vi "PMT_plus_Kinesis_plus_Keithley.vi"() -> ()   [LabVIEW 2022 SP3]
uses:
  <vilib>/Utility/file.llb/Write Delimited Spreadsheet (string).vi
  <vilib>/Analysis/1siggen.llb/Ramp Pattern by Delta.vi
  <vilib>/Utility/file.llb/Write Delimited Spreadsheet (DBL).vi
  C:/Users/Public/OneDrive/Desktop/PMT program/SampleCodeLabView/Kinesis_with_LabVIEW_Examples_LV12 - v3/ThorLabs.MotionControl.KCube.DCServoCLI.dll
  Kinesis_with_LabVIEW_Examples_LV12 - v3/ThorLabs.MotionControl.KCube.DCServoCLI.dll
  <vilib>/Analysis/NI_AALBase.lvlib
  C:/Users/Public/OneDrive/Desktop/PMT program/SampleCodeLabView/Kinesis_with_LabVIEW_Examples_LV12 - v3/Thorlabs.MotionControl.Controls.dll
  Kinesis_with_LabVIEW_Examples_LV12 - v3/Thorlabs.MotionControl.Controls.dll
  test_save_lv22/Close.vi/Close Folder/Users/Public/OneDrive/Desktop/Keithley_2450_2470_1_4_0_LV2015_NewReadme2_2450-LV2015-1.4.0/Keithley 2450/Keithley 2450.lvlib
  D:/Download/Keithley 24XX/Keithley 24XX Folder/D/Download/Keithley 24XX/Keithley 24XX.lvlib
panel:
  out "current 2410":dbl format="%e"
  in  "top: 2450\nbottom: 2410":bool
  in  "VISA resource name 2410":refnum<visa-resource-name>="GPIB1::16::INSTR"
  in  "wait for cur meas":u32=100
  out "XY Graph":cluster{dbl[], dbl[]}(graph)
  out "mean":dbl=49.0
  out "standard deviation":dbl
  out "OLD":bool
  out "data":u32[](array[numeric])=[49, 49]
  out "Actual Voltage":dbl
  out "current":dbl=2.5622937e-12 format="%e"
  out "error out":errorcluster
  out "Set Voltage":dbl
  in  "VISA resource name 2450":refnum<visa-resource-name>="GPIB0::1::INSTR"
  in  "error in (no error)":errorcluster
  out "Serial Configuration":T1={"Baud Rate"=9600, "Parity"=0, "Data Bits"=8, "Stop Bits"=10, "Flow Control"=0} {"Flow Control" items=["None", "XON/XOFF", "RTS/CTS", "XON/XOFF & RTS/CTS", "DTR/DSR", "XON/XOFF & DTR/DSR"]; "Stop Bits" items=["1.0"=10, "1.5"=15, "2.0"=20]; "Data Bits" items=["7"=7, "8"=8]; "Parity" items=["None", "Odd", "Even", "Mark", "Space"]; "Baud Rate" items=["300"=300, "600"=600, "1200"=1200, "2400"=2400, "4800"=4800, "9600"=9600, "19200"=19200]}
  in  "Num Current Meas":i32=20
  in  "Source Limit Level (0.1)":dbl=1e-08
  in  "wait for move (ms)":u32=14000
  out "Handle Number":i32=173123648
  in  "Start V":dbl format="%#_13g"
  in  "End V":dbl=0.2 format="%#_13g"
  in  "Step Size (V)":dbl=0.1 format="%#_13g"
  in  "Path":path=path "C:/Users/Public/OneDrive/Desktop/test.txt"
  in  "Use PMT?":bool=TRUE
  in  "Loop?":bool
  in  "KCubeDCServoControl":refnum<k24>(container)
  in  "Motor Controller SerialNumber":string="27268499"
  in  "quarter waveplate p1":dbl=142.0 format="%#_13g"
  in  "quarter waveplate p2":dbl=232.0 format="%#_13g"
  out "PC":dbl caption="Current Rotation Position"
  out "DB":u32[](array[numeric])=[49, 0, 0, 0, 0, 0, 0, 0, 0, 0, 0, 0, 0, 0, 0, 0]
  out "Overload":i32
  out "Gate Number":i32=1
  out "Num Gates Read":i32=2
  out "Gate Time Read":i32=100 caption="Gate time Read"
  out "Num Gates Set":i32=20
  out "Gate Time Set":i32=300
  out "PowerD":i32 caption="Power\nRead Data"
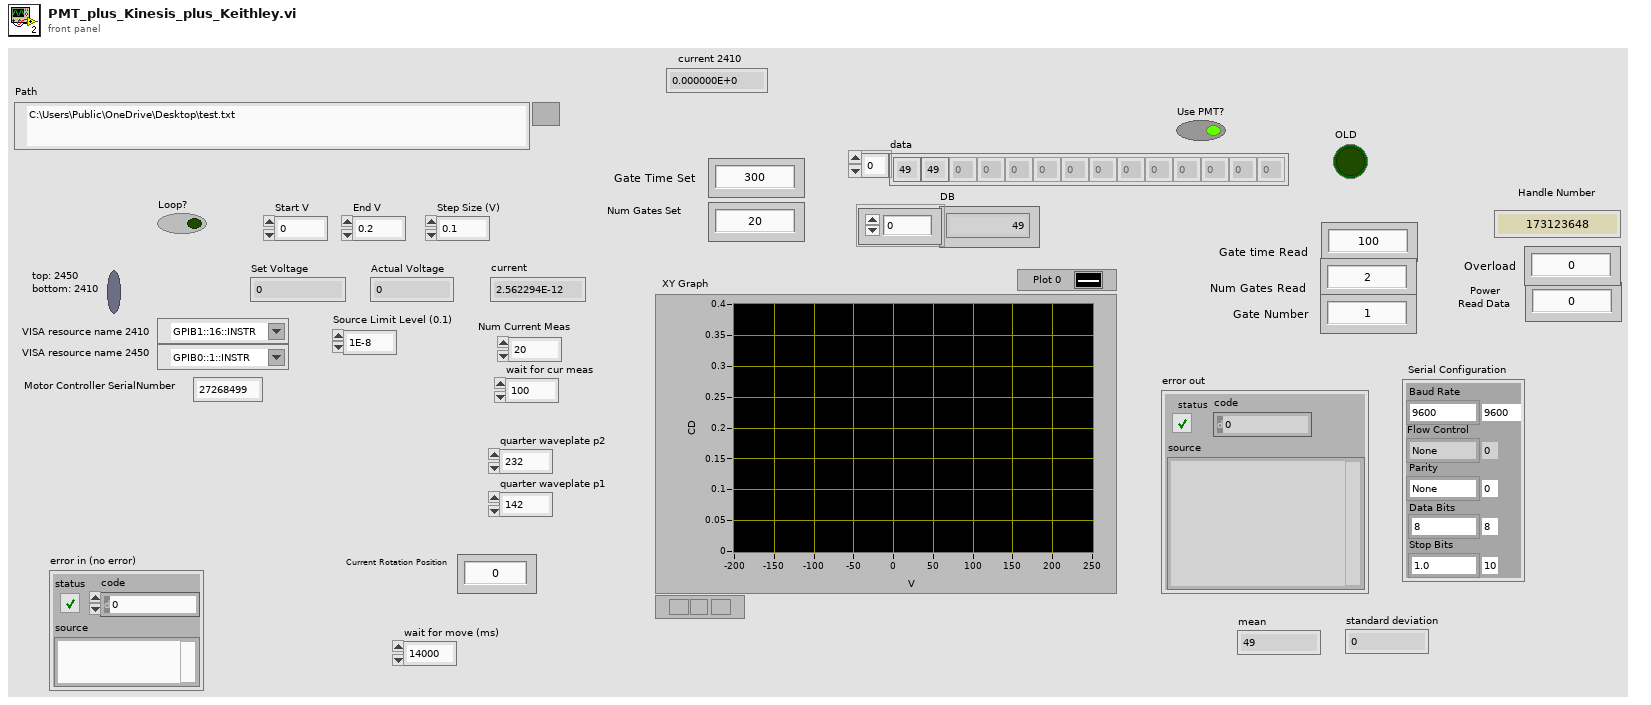
[diagram p1: front panel]
types:
  T1 = cluster{"Baud Rate":u32, "Parity":u16, "Data Bits":u16, "Stop Bits":u16, "Flow Control":u16}
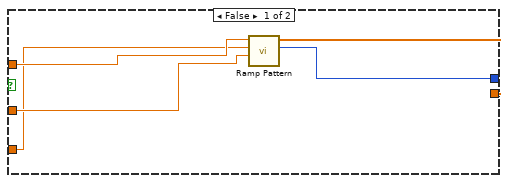
[diagram p2: hidden frame]
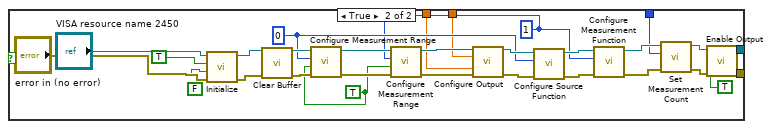
[diagram p3: hidden frame]
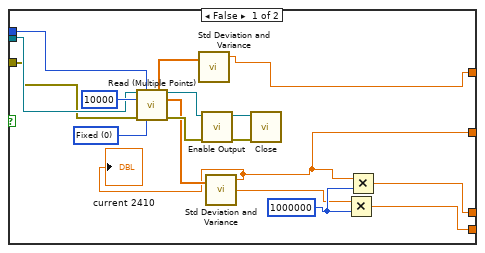
[diagram p4: hidden frame]
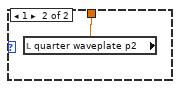
[diagram p5: hidden frame]
diagram:
  n1 = flat-sequence {
    tunnel: [w47] -> w22
    tunnel: [w38] -> w21
    tunnel: ["Path"] -> w20
    tunnel: [w37] -> w19
    tunnel: [w26] -> w18
    tunnel: [w23] -> w17
    tunnel: w22 -> [w83]
    tunnel: [w83] -> w16
    tunnel: w21 -> [w82]
    tunnel: [w82] -> w15
    tunnel: w20 -> [w81]
    tunnel: [w81] -> w14
    tunnel: w19 -> [w80]
    tunnel: [w80] -> w13
    tunnel: [w79] -> w12
    tunnel: w18 -> [w79]
    tunnel: ["wait for move (ms)"] -> w11
    tunnel: [w77] -> w10
    tunnel: w17 -> [w77]
    tunnel: w16 -> [w94]
    tunnel: [w94] -> w9
    tunnel: w15 -> [w93]
    tunnel: [w93] -> w8
    tunnel: w14 -> [w92]
    tunnel: [w92] -> w7
    tunnel: w13 -> [w91]
    tunnel: [w91] -> w6
    tunnel: w12 -> [w90]
    tunnel: [w89] -> w5
    tunnel: [w85] -> w4
    tunnel: w11 -> [w85]
    tunnel: [w84] -> w3
    tunnel: w10 -> [w84]
    tunnel: w9 -> [w106]
    tunnel: w8 -> [w105]
    tunnel: [w104] -> w2
    tunnel: w7 -> [w103]
    tunnel: w6 -> [w98]
    tunnel: w5 -> [w95]
    tunnel: w4 -> [w97]
    tunnel: w3 -> [w96]
    tunnel: [w95] -> w1
    tunnel: w2 -> [w644]
    tunnel: w1 -> [w637]
    frame #0 {
      # "open PMT and turn on power"
      n2 = local write "quarter waveplate p2"("quarter waveplate p2") -> ()
      n3 = local write "quarter waveplate p1"("quarter waveplate p1") -> ()
      n4 = call "Open.vi"("Serial Number"="30430219") -> ("Handle Number"=w51:i32)  [unwired: 9 in, 1 out]
      "Handle Number" <- w51
      n5 = case shown="True" "Loop?" {
        tunnel: "Start V" -> [w58 w69]
        tunnel: "End V" -> [w57 w67]
        tunnel: [w60 w66] -> w37
        tunnel: [w61 w65] -> w38
        tunnel: "Step Size (V)" -> [w59 w63]
        frame False {
          n6 = call-poly <vilib>:"Ramp Pattern.vi"("start"=w58, "end"=w57, "delta"=w59) -> ("samples"=w61:i32, "Ramp Pattern"=w60:dbl[])  [unwired: 6 in, 1 out]
        }
        frame True {
          w64 = -1.0
          n7 = Multiply(x=w63, y=w64) -> (x*y=w62:dbl)
          n8 = Multiply(x=w67, y=w64) -> (x*y=w68:dbl)
          n9 = call-poly <vilib>:"Ramp Pattern.vi"("start"=w69, "end"=w67, "delta"=w63) -> ("samples"=w73:i32, "Ramp Pattern"=w70:dbl[])  [unwired: 6 in, 1 out]
          n10 = call-poly <vilib>:"Ramp Pattern.vi"("start"=w68, "end"=w69, "delta"=w63) -> ("samples"=w76:i32, "Ramp Pattern"=w72:dbl[])  [unwired: 6 in, 1 out]
          n11 = call-poly <vilib>:"Ramp Pattern.vi"("start"=w67, "end"=w68, "delta"=w62) -> ("samples"=w74:i32, "Ramp Pattern"=w71:dbl[])  [unwired: 6 in, 1 out]
          n12 = Add(x=w73, y=w74) -> (x+y=w75:i32)
          n13 = Build Array (concatenate)(w70, w71, w72) -> (w66:dbl[])
          n14 = Add(x=w75, y=w76) -> (x+y=w65:i32)
        }
      }
      n15 = call "Read HV.vi"("handle"=w51) -> ("HV out"=w50:i32, "handle out"=w54:i32)  [unwired: 8 in, 1 out]
      n16 = Boolean To (0,1)(Boolean="Use PMT?") -> (0, 1=w52:i16)
      n17 = local write "PowerD"(w50) -> ()
      n18 = To Long Integer(number=w52) -> (32bit integer=w53:i32)
      n19 = call "Set HV.vi"("HV"=w53, "handle"=w54) -> ("handle out"=w56:i32)  [unwired: 8 in, 1 out]
      n20 = property class="KCubeDCServoControl"(reference="KCubeDCServoControl", "SerialNumber"="Motor Controller SerialNumber") -> (reference out=w36:refnum<k24>)  [unwired: 1 in, 1 out]
      n21 = invoke class="KCubeDCServoControl" method="CreateDevice"(reference=w36) -> (reference out=w33:refnum<k24>)  [unwired: 2 in, 2 out]
      n22 = property class="KCubeDCServoControl"(reference=w33) -> ("Device"=w23:refnum<k24>)  [unwired: 1 in, 2 out]
      n23 = call "Read HV.vi"("handle"=w56) -> ("HV out"=w55:i32, "handle out"=w47:i32)  [unwired: 8 in, 1 out]
      n24 = local write "PowerD"(w55) -> ()
      n25 = invoke class="KCubeDCServo" method="GetPositionCounter"(reference=w23) -> (reference out=w29:refnum<k24>, "GetPositionCounter"=w32:i32)  [unwired: 2 in, 1 out]
      n26 = Divide(x=w32, y=1919.6418578623338) -> (x/y=w30:dbl)
      n27 = local write "PC"(w30) -> ()
      n28 = invoke class="KCubeDCServo" method="SetMoveAbsolutePosition"(reference=w29, "position"="quarter waveplate p1") -> (reference out=w28:refnum<k24>)  [unwired: 2 in, 3 out]
      n29 = invoke class="KCubeDCServo" method="MoveAbsolute"(reference=w28, "waitTimeout"=0) -> (reference out=w26:refnum<k24>)  [unwired: 2 in, 3 out]
      n30 = Build Array("# SetVoltage(V) ActualVoltage(V) CountsMeancirc1 Countsmeancirc2 CountsStdcirc1 CountsStdcirc2 Current(uA) CurrentStd(uA) CircularDichroism") -> (w42:string[])
      n31 = call-poly <vilib>:"Write Delimited Spreadsheet.vi"("file path (dialog if empty)"="Path", "1D data"=w42, "append to file? (new file:F)"=TRUE) -> ()  [unwired: 11 in, 2 out]
    }
    frame #1 {
      n32 = Wait (ms)(milliseconds to wait="wait for move (ms)") -> ()  [unwired: 1 out]
    }
    frame #2 {
      n33 = invoke class="KCubeDCServo" method="GetPositionCounter"(reference=w90) -> (reference out=w89:refnum<k24>, "GetPositionCounter"=w87:i32)  [unwired: 2 in, 1 out]
      n34 = Divide(x=w87, y=1919.6418578623338) -> (x/y=w86:dbl)
      n35 = local write "PC"(w86) -> ()
    }
    frame #3 {
      w101 = 0
      w102 = 0
      n36 = Initialize Array(w102, w102) -> (w99:i32[])
      n37 = Initialize Array(w101, w101) -> (w100:i32[])
      n38 = for {
        N: w105 -> [_]
        tunnel: w98 -> [w162] mode=indexing
        tunnel: w106 -> [w138]
        tunnel: [w161] -> w104
        tunnel: w103 -> [w134]
        shift-right: [w152] -> _
        shift-left: w99 -> [w157]
        shift-right: [w153] -> _
        shift-left: w100 -> [w156]
        tunnel: w95 -> [w130]
        tunnel: w97 -> [w126]
        tunnel: w96 -> [w112]
        n39 = flat-sequence {
          tunnel: w156 -> [w169]
          tunnel: w157 -> [w174]
          tunnel: w162 -> [w168]
          tunnel: [w168] -> w151
          tunnel: [w174] -> w149
          tunnel: [w169] -> w147
          tunnel: [w167] -> w145
          tunnel: [w166] -> w143
          tunnel: ["Num Current Meas"] -> w139
          tunnel: w138 -> [w173]
          tunnel: [w173] -> w135
          tunnel: w134 -> [w172]
          tunnel: [w172] -> w131
          tunnel: w130 -> [w171]
          tunnel: [w171] -> w127
          tunnel: w112 -> [w170]
          tunnel: [w170] -> w110
          tunnel: ["top: 2450\nbottom: 2410"] -> w107
          tunnel: w151 -> [w233]
          tunnel: [w233] -> w150
          tunnel: w149 -> [w232]
          tunnel: [w232] -> w148
          tunnel: w147 -> [w231]
          tunnel: [w231] -> w146
          tunnel: w145 -> [w230]
          tunnel: [w230] -> w144
          tunnel: w143 -> [w229]
          tunnel: [w229] -> w142
          tunnel: [w228] -> w140
          tunnel: w139 -> [w228]
          tunnel: [w226] -> w136
          tunnel: w135 -> [w226]
          tunnel: [w225] -> w132
          tunnel: w131 -> [w225]
          tunnel: [w224] -> w128
          tunnel: w127 -> [w224]
          tunnel: [w223] -> w111
          tunnel: w110 -> [w223]
          tunnel: [w222] -> w108
          tunnel: w107 -> [w222]
          tunnel: [w248] -> w160
          tunnel: [w235] -> w159
          tunnel: [w241] -> w158
          tunnel: [w247] -> w155
          tunnel: [w246] -> w154
          tunnel: w150 -> [w248]
          tunnel: w148 -> [w247]
          tunnel: w146 -> [w246]
          tunnel: w144 -> [w244]
          tunnel: w142 -> [w245]
          tunnel: [w242] -> w141
          tunnel: w140 -> [w243]
          tunnel: [w239] -> w137
          tunnel: w136 -> [w239]
          tunnel: [w238] -> w133
          tunnel: w132 -> [w238]
          tunnel: [w237] -> w129
          tunnel: w128 -> [w237]
          tunnel: w111 -> [w236]
          tunnel: [w236] -> w109
          tunnel: w108 -> [w234]
          tunnel: w160 -> [w314]
          tunnel: w159 -> [w313]
          tunnel: w158 -> [w312]
          tunnel: w155 -> [w311]
          tunnel: w154 -> [w310]
          tunnel: [w315] -> w125
          tunnel: [w309] -> w122
          tunnel: w141 -> [w308]
          tunnel: w137 -> [w307]
          tunnel: w133 -> [w303]
          tunnel: w129 -> [w305]
          tunnel: w126 -> [w304]
          tunnel: [w303] -> w120
          tunnel: [w302] -> w119
          tunnel: [w297] -> w118
          tunnel: [w296] -> w117
          tunnel: [w295] -> w116
          tunnel: [w294] -> w115
          tunnel: [w293] -> w114
          tunnel: [w292] -> w113
          tunnel: w109 -> [w291]
          tunnel: w125 -> [w631]
          tunnel: [w631] -> w124
          tunnel: [w622] -> w123
          tunnel: w122 -> [w613]
          tunnel: [w612] -> w121
          tunnel: w120 -> [w629]
          tunnel: w119 -> [w627]
          tunnel: w118 -> [w610]
          tunnel: w117 -> [w620]
          tunnel: w116 -> [w626]
          tunnel: w115 -> [w625]
          tunnel: w114 -> [w623]
          tunnel: w113 -> [w621]
          tunnel: [w633] -> w152
          tunnel: [w634] -> w153
          tunnel: [w635] -> w161
          tunnel: w124 -> [w635]
          tunnel: w123 -> [w634]
          tunnel: w121 -> [w633]
          frame #0 {
            n40 = case shown="False" "top: 2450\nbottom: 2410" {
              tunnel: w168 -> [w175 w198]
              tunnel: [w177 w196] -> w167
              tunnel: [w178 w195] -> w166
              tunnel: "Num Current Meas" -> [_ w194]
              tunnel: "Source Limit Level (0.1)" -> [w176 w193]
              frame False {
                w180 = TRUE
                w181 = u16 0 items=["Voltage", "Current"] ("Source Mode  (0: Voltage)")
                w182 = u16 1 items=["Volts", "Current", "Resistance"] ("Function (0: Volts)")
                w183 = u16 0 items=["Volts", "Current", "Resistance"] ("Function (0: Volts)")
                n41 = call "Initialize.vi"("Reset (True)"=FALSE, "VISA resource name"="VISA resource name 2410") -> ("error out"=w190:errorcluster, "VISA resource name out"=w191:refnum<visa-resource-name>)  [unwired: 8 in]
                n42 = call "Configure Measurement.vi"("error in (no error)"=w190, "Enable Auto Range (T:Enable)"=w180, "Function (0: Volts)"=w183, "VISA resource name"=w191) -> ("error out"=w189:errorcluster, "VISA resource name out"=w188:refnum<visa-resource-name>)  [unwired: 6 in]
                n43 = call "Configure Measurement.vi"("error in (no error)"=w189, "Enable Auto Range (T:Enable)"=w180, "Function (0: Volts)"=w182, "VISA resource name"=w188) -> ("error out"=w186:errorcluster, "VISA resource name out"=w187:refnum<visa-resource-name>)  [unwired: 6 in]
                n44 = call "Configure Output.vi"("Source Mode  (0: Voltage)"=w181, "error in (no error)"=w186, "Compliance  Level (0.1)"=w176, "Output Level (0)"=w175, "VISA resource name"=w187) -> ("error out"=w184:errorcluster, "VISA resource name out"=w185:refnum<visa-resource-name>)  [unwired: 5 in]
                n45 = call "Enable Output.vi"("error in (no error)"=w184, "VISA resource name"=w185) -> ("error out"=w177:errorcluster, "VISA resource name out"=w178:refnum<visa-resource-name>)  [unwired: 8 in]
              }
              frame True {
                w197 = 1
                w200 = 0
                w201 = TRUE
                n46 = call "Initialize.vi"("error in (no error)"="error in (no error)", "Reset (True)"=FALSE, "ID Query (True)"=TRUE, "VISA resource name"="VISA resource name 2450") -> ("error out"=w221:errorcluster, "VISA resource name out"=w218:refnum<visa-resource-name>)  [unwired: 6 in]
                n47 = call "Clear Buffer.vi"("VISA resource name"=w218, "error in (no error)"=w221) -> ("VISA resource name out"=w213:refnum<visa-resource-name>, "error out"=w212:errorcluster)  [unwired: 12 in]
                n48 = call "Configure Measurement Range.vi"("error in (no error)"=w212, "Enable Auto Range (T:Enable)"=w201, "Function (0: Volts)"=w200, "VISA resource name"=w213) -> ("error out"=w204:errorcluster, "VISA resource name out"=w205:refnum<visa-resource-name>)  [unwired: 6 in]
                n49 = call "Configure Measurement Range.vi"("error in (no error)"=w204, "Enable Auto Range (T:Enable)"=w201, "Function (0: Volts)"=w197, "VISA resource name"=w205) -> ("error out"=w208:errorcluster, "VISA resource name out"=w211:refnum<visa-resource-name>)  [unwired: 6 in]
                n50 = call "Configure Output.vi"("VISA resource name"=w211, "Source Level (0)"=w198, "Source Limit Level (0.1)"=w193, "error in (no error)"=w208) -> ("VISA resource name out"=w210:refnum<visa-resource-name>, "error out"=w207:errorcluster)  [unwired: 10 in]
                n51 = call "Configure Source Function.vi"("error in (no error)"=w207, "Function (0: Volts)"=w200, "VISA resource name"=w210) -> ("error out"=w206:errorcluster, "VISA resource name out"=w209:refnum<visa-resource-name>)  [unwired: 7 in]
                n52 = call "Configure Measurement Function.vi"("error in (no error)"=w206, "Function (0: Volts)"=w197, "VISA resource name"=w209) -> ("error out"=w217:errorcluster, "VISA resource name out"=w214:refnum<visa-resource-name>)  [unwired: 7 in]
                n53 = call "Set Measurement Count.vi"("error in (no error)"=w217, "Measurement Count (1)"=w194, "VISA resource name"=w214) -> ("error out"=w216:errorcluster, "VISA resource name out"=w215:refnum<visa-resource-name>)  [unwired: 7 in]
                n54 = call "Enable Output.vi"("error in (no error)"=w216, "Enable Output (T: Enable)"=TRUE, "VISA resource name"=w215) -> ("error out"=w196:errorcluster, "VISA resource name out"=w195:refnum<visa-resource-name>)  [unwired: 7 in]
              }
            }
            "Set Voltage" <- w168
          }
          frame #1 {
            n55 = Wait (ms)(milliseconds to wait="wait for cur meas") -> ()  [unwired: 1 out]
          }
          frame #2 {
            n56 = case shown="True" w234 {
              tunnel: w245 -> [w251 w290]
              tunnel: w244 -> [w249 w289]
              tunnel: w243 -> [w250 w288]
              tunnel: [w252 w287] -> w242
              tunnel: [w253 w286] -> w241
              tunnel: [w254 w271] -> w240
              tunnel: [w257 w266] -> w235
              frame False {
                w256 = 1000000
                w265 = u16 0 items=["Fixed", "Sweep", "List"] ("Output Mode (0: Fixed)")
                n57 = call "Read (Multiple Points).vi"("VISA resource name"=w251, "Sample Count (1)"=w250, "Timeout (10000 ms)"=10000, "error in (no error)"=w249, "Output Mode (0: Fixed)"=w265) -> ("Voltage"=w258:sgl[], "VISA resource name out"=w263:refnum<visa-resource-name>, "Current"=w259:sgl[], "error out"=w260:errorcluster)  [unwired: 4 in, 3 out]
                n58 = call <vilib>:"Std Deviation and Variance.vi"("X"=w258) -> ("mean"=w257:dbl)  [unwired: 1 in, 2 out]
                n59 = call "Enable Output.vi"("error in (no error)"=w260, "VISA resource name"=w263) -> ("error out"=w261:errorcluster, "VISA resource name out"=w262:refnum<visa-resource-name>)  [unwired: 8 in]
                n60 = call <vilib>:"Std Deviation and Variance.vi"("X"=w259) -> ("mean"=w254:dbl, "standard deviation"=w255:dbl)  [unwired: 1 in, 1 out]
                "current 2410" <- w254
                n61 = call "Close.vi"("error in (no error)"=w261, "VISA resource name"=w262) -> ()  [unwired: 9 in, 1 out]
                n62 = Multiply(x=w255, y=w256) -> (x*y=w252:dbl)
                n63 = Multiply(x=w254, y=w256) -> (x*y=w253:dbl)
              }
              frame True {
                w270 = 1000000
                n64 = call "Make Reading and Store in Buffer.vi"("VISA resource name"=w290, "error in (no error)"=w289) -> ("VISA resource name out"=w282:refnum<visa-resource-name>, "error out"=w281:errorcluster)  [unwired: 12 in]
                n65 = call "Read (Multiple Points).vi"("VISA resource name"=w282, "Start Index (1)"=u32 1, "End Index (1)"=w288, "error in (no error)"=w281) -> ("VISA resource name out"=w274:refnum<visa-resource-name>, "Data out"=w279:string, "error out"=w273:errorcluster)  [unwired: 9 in]
                n66 = Spreadsheet String To Array(delimiter (Tab)=",", format string="%s", spreadsheet string=w279, array type (2D Dbl)=dbl[] []) -> (array=w275:dbl[])
                n67 = call "Get Source Level.vi"("error in (no error)"=w273, "VISA resource name"=w274) -> ("error out"=w284:errorcluster, "Voltage Level Out"=w266:dbl, "VISA resource name out"=w285:refnum<visa-resource-name>)  [unwired: 6 in, 1 out]
                n68 = call <vilib>:"Std Deviation and Variance.vi"("X"=w275) -> ("mean"=w271:dbl, "standard deviation"=w272:dbl)  [unwired: 1 in, 1 out]
                n69 = call "Enable Output.vi"("error in (no error)"=w284, "Enable Output (T: Enable)"=TRUE, "VISA resource name"=w285) -> ("error out"=w267:errorcluster, "VISA resource name out"=w268:refnum<visa-resource-name>)  [unwired: 7 in]
                n70 = Multiply(x=w272, y=w270) -> (x*y=w287:dbl)
                n71 = Multiply(x=w271, y=w270) -> (x*y=w286:dbl)
                n72 = call "Close.vi"("error in (no error)"=w267, "VISA resource name"=w268) -> ("error out"=→"error out":errorcluster)  [unwired: 9 in]
              }
            }
            "current" <- w240
            "Actual Voltage" <- w235
          }
          frame #3 {
            w299 = 0
            w301 = 0
            n73 = Initialize Array(w301, w301) -> (w300:i32[])
            n74 = Initialize Array(w299, w299) -> (w298:i32[])
            n75 = for {
              N: 2 -> [_]
              tunnel: w314 -> [w425]
              tunnel: w313 -> [w424]
              tunnel: w312 -> [w423]
              tunnel: w311 -> [w345]
              tunnel: w310 -> [w422]
              tunnel: [w421] -> w309
              tunnel: w308 -> [w420]
              shift-right: [w426] -> w315
              shift-left: w307 -> [w419]
              tunnel: w305 -> [w357]
              tunnel: w304 -> [w356]
              tunnel: [w346] -> w302
              shift-right: [w324] -> w297
              shift-left: w300 -> [w344]
              shift-right: [w323] -> w296
              shift-left: w298 -> [w334]
              tunnel: [w322] -> w295
              tunnel: [w321] -> w294
              tunnel: [w320] -> w293
              tunnel: [w319] -> w292
              tunnel: w291 -> [w318]
              i -> [w355]
              (unwired) "# SetVoltage2450(V) ActualVoltage2450(V) CountsMean CountsStd Current2450(uA) Current2450Std(uA)"
              # "- actual voltage array\n- actual voltage current\n- set voltage current\n-  current current\n- current std current"
              n76 = flat-sequence {
                tunnel: [w438] -> w371
                tunnel: [w436] -> w369
                tunnel: [w437] -> w367
                tunnel: w425 -> [w438]
                tunnel: w424 -> [w437]
                tunnel: w423 -> [w436]
                tunnel: w345 -> [w435]
                tunnel: [w435] -> w365
                tunnel: w422 -> [w434]
                tunnel: [w434] -> w363
                tunnel: w420 -> [w433]
                tunnel: [w433] -> w361
                tunnel: w419 -> [w432]
                tunnel: [w432] -> w359
                tunnel: w357 -> [_]
                tunnel: w355 -> [w430]
                tunnel: w344 -> [w429]
                tunnel: [w429] -> w340
                tunnel: w334 -> [w428]
                tunnel: [w428] -> w327
                tunnel: w318 -> [w427]
                tunnel: [w427] -> w317
                tunnel: w371 -> [w452]
                tunnel: [w452] -> w370
                tunnel: w369 -> [w451]
                tunnel: [w451] -> w368
                tunnel: w367 -> [w450]
                tunnel: [w450] -> w366
                tunnel: w365 -> [w449]
                tunnel: [w449] -> w364
                tunnel: w363 -> [w448]
                tunnel: [w448] -> w362
                tunnel: w361 -> [w447]
                tunnel: [w447] -> w360
                tunnel: w359 -> [w446]
                tunnel: [w446] -> w358
                tunnel: [w444] -> w341
                tunnel: w340 -> [w444]
                tunnel: [w443] -> w328
                tunnel: w327 -> [w443]
                tunnel: w317 -> [w442]
                tunnel: [w441] -> w316
                tunnel: [w460] -> w418
                tunnel: [w466] -> w417
                tunnel: w370 -> [w466]
                tunnel: [w465] -> w416
                tunnel: w368 -> [w465]
                tunnel: [w464] -> w415
                tunnel: w366 -> [w464]
                tunnel: [w463] -> w414
                tunnel: w364 -> [w463]
                tunnel: [w462] -> w413
                tunnel: w362 -> [w462]
                tunnel: [w461] -> w412
                tunnel: w360 -> [w461]
                tunnel: w358 -> [w460]
                tunnel: w356 -> [w459]
                tunnel: [w458] -> w342
                tunnel: w341 -> [w458]
                tunnel: [w457] -> w329
                tunnel: w328 -> [w457]
                tunnel: w316 -> [w453]
                tunnel: w418 -> [w481]
                tunnel: [w476] -> w411
                tunnel: [w474] -> w410
                tunnel: w417 -> [w474]
                tunnel: [w473] -> w409
                tunnel: w416 -> [w473]
                tunnel: [w472] -> w408
                tunnel: w415 -> [w472]
                tunnel: [w471] -> w407
                tunnel: w414 -> [w471]
                tunnel: [w470] -> w406
                tunnel: w413 -> [w470]
                tunnel: [w469] -> w405
                tunnel: w412 -> [w469]
                tunnel: [w468] -> w343
                tunnel: w342 -> [w468]
                tunnel: [w467] -> w330
                tunnel: w329 -> [w467]
                tunnel: [w492] -> w404
                tunnel: w411 -> [w494]
                tunnel: [w489] -> w403
                tunnel: w410 -> [w489]
                tunnel: w409 -> [w488]
                tunnel: [w488] -> w402
                tunnel: [w487] -> w401
                tunnel: w408 -> [w487]
                tunnel: [w486] -> w400
                tunnel: w407 -> [w486]
                tunnel: [w485] -> w399
                tunnel: w406 -> [w485]
                tunnel: [w484] -> w398
                tunnel: w405 -> [w484]
                tunnel: w343 -> [w483]
                tunnel: [w483] -> w337
                tunnel: [w482] -> w331
                tunnel: w330 -> [w482]
                tunnel: w404 -> [w509]
                tunnel: [w509] -> w397
                tunnel: [w505] -> w396
                tunnel: [w505] -> w395
                tunnel: [w504] -> w394
                tunnel: w403 -> [w504]
                tunnel: [w503] -> w393
                tunnel: w402 -> [w503]
                tunnel: w401 -> [w502]
                tunnel: [w502] -> w392
                tunnel: [w501] -> w391
                tunnel: w400 -> [w501]
                tunnel: [w500] -> w390
                tunnel: w399 -> [w500]
                tunnel: w398 -> [w499]
                tunnel: [w499] -> w389
                tunnel: [w498] -> w338
                tunnel: w337 -> [w498]
                tunnel: [w497] -> w332
                tunnel: w331 -> [w497]
                tunnel: w397 -> [w524]
                tunnel: [w520] -> w388
                tunnel: w396 -> [w519]
                tunnel: w395 -> [w518]
                tunnel: [w519] -> w387
                tunnel: [w518] -> w386
                tunnel: w394 -> [w517]
                tunnel: [w517] -> w385
                tunnel: [w516] -> w384
                tunnel: w393 -> [w516]
                tunnel: [w515] -> w383
                tunnel: w392 -> [w515]
                tunnel: [w514] -> w382
                tunnel: w391 -> [w514]
                tunnel: [w513] -> w381
                tunnel: w390 -> [w513]
                tunnel: [w512] -> w380
                tunnel: w389 -> [w512]
                tunnel: [w511] -> w339
                tunnel: w338 -> [w511]
                tunnel: [w510] -> w333
                tunnel: w332 -> [w510]
                tunnel: [w539] -> w379
                tunnel: w388 -> [w538]
                tunnel: w387 -> [w537]
                tunnel: w386 -> [w536]
                tunnel: [w535] -> w378
                tunnel: [w532] -> w377
                tunnel: w385 -> [w532]
                tunnel: [w531] -> w376
                tunnel: w384 -> [w531]
                tunnel: w383 -> [w530]
                tunnel: [w530] -> w375
                tunnel: [w529] -> w374
                tunnel: w382 -> [w529]
                tunnel: [w528] -> w373
                tunnel: w381 -> [w528]
                tunnel: [w527] -> w372
                tunnel: w380 -> [w527]
                tunnel: w339 -> [w526]
                tunnel: [w526] -> w336
                tunnel: w333 -> [w525]
                tunnel: [w525] -> w326
                tunnel: w379 -> [w595]
                tunnel: [w594] -> w353
                tunnel: [w593] -> w354
                tunnel: w378 -> [w593]
                tunnel: w377 -> [w592]
                tunnel: [w592] -> w352
                tunnel: [w591] -> w351
                tunnel: w376 -> [w591]
                tunnel: [w590] -> w350
                tunnel: w375 -> [w590]
                tunnel: [w589] -> w349
                tunnel: w374 -> [w589]
                tunnel: w373 -> [w588]
                tunnel: [w588] -> w348
                tunnel: [w587] -> w347
                tunnel: w372 -> [w587]
                tunnel: w336 -> [w586]
                tunnel: [w586] -> w335
                tunnel: w326 -> [w585]
                tunnel: [w585] -> w325
                tunnel: [w609] -> w426
                tunnel: w353 -> [w609]
                tunnel: w352 -> [w607]
                tunnel: w351 -> [w601]
                tunnel: w350 -> [w599]
                tunnel: w349 -> [w596]
                tunnel: w348 -> [w600]
                tunnel: [w596] -> w421
                tunnel: w347 -> [w598]
                tunnel: w354 -> [w608]
                tunnel: [w607] -> w346
                tunnel: w335 -> [w606]
                tunnel: w325 -> [w605]
                tunnel: [w603] -> w324
                tunnel: [w602] -> w323
                tunnel: [w601] -> w322
                tunnel: [w598] -> w321
                tunnel: [w600] -> w320
                tunnel: [w599] -> w319
                frame #0 {
                  n77 = case shown="0, Default" w430 {
                    tunnel: [w439 w440] -> w431
                    frame 0, Default {
                      n78 = local read "quarter waveplate p1"() -> (w439:dbl)
                    }
                    frame 1 {
                      n79 = local read "quarter waveplate p2"() -> (w440:dbl)
                    }
                  }
                  n80 = invoke class="KCubeDCServo" method="SetMoveAbsolutePosition"(reference=w427, "position"=w431) -> ()  [unwired: 2 in, 4 out]
                }
                frame #1 {
                  n81 = invoke class="KCubeDCServo" method="MoveAbsolute"(reference=w442, "waitTimeout"=0) -> (reference out=w441:refnum<k24>)  [unwired: 2 in, 3 out]
                }
                frame #2 {
                  n82 = Wait (ms)(milliseconds to wait=w459) -> ()  [unwired: 1 out]
                  n83 = invoke class="KCubeDCServo" method="GetPositionCounter"(reference=w453) -> ("GetPositionCounter"=w455:i32)  [unwired: 2 in, 2 out]
                  n84 = Divide(x=w455, y=1919.6418578623338) -> (x/y=w454:dbl)
                  n85 = local write "PC"(w454) -> ()
                }
                frame #3 {
                  # "set gate time"
                  n86 = local read "Gate Time Set"() -> (w478:i32)
                  n87 = Wait (ms)(milliseconds to wait=u32 200) -> ()  [unwired: 1 out]
                  n88 = To Long Integer(number=w478) -> (32bit integer=w479:i32)
                  n89 = call "Set IT.vi"("IT"=w479, "handle"=w481) -> ("handle out"=w480:i32)  [unwired: 8 in, 1 out]
                  n90 = call "Read IT.vi"("handle"=w480) -> ("IT out"=w477:i32, "handle out"=w476:i32)  [unwired: 8 in, 1 out]
                  n91 = local write "Gate Time Read"(w477) -> ()
                }
                frame #4 {
                  # "set number of gates"
                  n92 = local read "Num Gates Set"() -> (w496:i32)
                  n93 = Wait (ms)(milliseconds to wait=u32 200) -> ()  [unwired: 1 out]
                  n94 = To Long Integer(number=w496) -> (32bit integer=w495:i32)
                  n95 = call "Set RN.vi"("RN"=w495, "handle"=w494) -> ("handle out"=w493:i32)  [unwired: 8 in, 1 out]
                  n96 = call "Read RN.vi"("handle"=w493) -> ("RN out"=w491:i32, "handle out"=w492:i32)  [unwired: 8 in, 1 out]
                  n97 = local write "Num Gates Read"(w491) -> ()
                }
                frame #5 {
                  # "gate number data"
                  # "count data"
                  n98 = local write "Gate Number"(0) -> ()
                  n99 = Initialize Array(u32 0, 0 ("次元サイズ")) -> (w505:u32[])
                }
                frame #6 {
                  n100 = Boolean To (0,1)(Boolean=TRUE ("Correction")) -> (0, 1=w523:i16)
                  n101 = To Long Integer(number=w523) -> (32bit integer=w522:i32)
                  n102 = call "Count Start.vi"("Correction"=w522, "handle"=w524) -> ("handle out"=w520:i32)  [unwired: 8 in, 1 out]
                }
                frame #7 {
                  n103 = local read "Num Gates Read"() -> (w534:i32)
                  n104 = for {
                    N: w534 -> [_]
                    shift-right: [w540] -> w535
                    shift-left: w537 -> [w548]
                    shift-right: [w544] -> _
                    shift-left: w536 -> [w547]
                    tunnel: w538 -> [w549]
                    tunnel: [w550] -> w539
                    tunnel: [w540] -> w533
                    n105 = flat-sequence {
                      tunnel: [w560] -> w554
                      tunnel: [w559] -> w545
                      tunnel: [w558] -> w542
                      tunnel: w549 -> [w560]
                      tunnel: w548 -> [w559]
                      tunnel: w547 -> [w558]
                      tunnel: [w571] -> w553
                      tunnel: w554 -> [w570]
                      tunnel: [w565] -> w552
                      tunnel: [w564] -> w551
                      tunnel: [w563] -> w546
                      tunnel: w545 -> [w563]
                      tunnel: [w562] -> w543
                      tunnel: w542 -> [w562]
                      tunnel: [w561] -> w541
                      tunnel: w553 -> [w584]
                      tunnel: w552 -> [w579]
                      tunnel: w551 -> [w578]
                      tunnel: w546 -> [w576]
                      tunnel: w543 -> [w575]
                      tunnel: w541 -> [w574]
                      tunnel: [w584] -> w550
                      tunnel: [w577] -> w540
                      tunnel: [w572] -> w544
                      frame #0 {
                        n106 = Initialize Array(u32 0, 16 ("次元サイズ")) -> (w555:u32[])
                        n107 = local write "DB"(w555) -> ()
                      }
                      frame #1 {
                        # "read data"
                        n108 = local read "Gate Number"() -> (w569:i32)
                        n109 = local read "Overload"() -> (w568:i32)
                        n110 = local read "DB"() -> (w566:u32[])
                        n111 = call "Read Data.vi"("OLD"=w568, "DataBuf"=w566, "GateNum"=w569, "handle"=w570) -> ("OLD out"=w567:i32, "DataBuf out"=w564:u32[], "GateNum out"=w561:i32, "handle out"=w571:i32, "function return"=w565:u32)  [unwired: 3 in]
                        n112 = local write "Gate Number"(w561) -> ()
                        n113 = local write "DB"(w564) -> ()
                        n114 = local write "Overload"(w567) -> ()
                      }
                      frame #2 {
                        # "Pickup Tans Data!"
                        n115 = To Long Integer(number=w579) -> (32bit integer=w580:i32)
                        n116 = Build Array(w574) -> (w573:i32[])
                        n117 = local read "Overload"() -> (w582:i32)
                        n118 = Build Array (concatenate)(w575, w573) -> (w572:u32[])
                        n119 = Array Subset(array=w578, length=w580) -> (w581:u32[])  [unwired: 1 in]
                        n120 = Not Equal To 0?(x=w582) -> (x != 0?=→"OLD":bool)
                        n121 = Build Array (concatenate)(w576, w581) -> (w577:u32[])
                      }
                    }
                  }
                  "data" <- w533
                }
                frame #8 {
                  # "data"
                  n122 = call "Count Stop.vi"("handle"=w595) -> ("handle out"=w594:i32)  [unwired: 9 in, 1 out]
                }
                frame #9 {
                  n123 = call <vilib>:"Std Deviation and Variance.vi"("X"=w608) -> ("mean"=w597:dbl, "standard deviation"=w604:dbl)  [unwired: 1 in, 1 out]
                  "mean" <- w597
                  "standard deviation" <- w604
                  n124 = Build Array (concatenate)(w605, w604) -> (w602:dbl[])
                  n125 = Build Array (concatenate)(w606, w597) -> (w603:dbl[])
                }
              }
            }
          }
          frame #4 {
            (unwired) "# SetVoltage2450(V) ActualVoltage2450(V) CountsMeanCirc1 CountsMeanCirc2 CountsStdCirc1 CountsStdCirc2 Current2450(uA) Current2450Std(uA)\nCirculardichroism"
            n126 = Build Array (concatenate)(w623, w621) -> (w622:dbl[])
            n127 = Index Array(array=w610, index=1) -> (element=w616:dbl)
            n128 = Index Array(array=w610, index=0) -> (element=w617:dbl)
            n129 = Subtract(x=w617, y=w616) -> (x-y=w615:dbl)
            n130 = Add(x=w617, y=w616) -> (x+y=w614:dbl)
            n131 = Divide(x=w615, y=w614) -> (x/y=w611:dbl)
            n132 = Build Array (concatenate)(w627, w621, w610, w620, w626, w625, w611) -> (w624:dbl[])
            n133 = call-poly <vilib>:"Write Delimited Spreadsheet.vi"("file path (dialog if empty)"=w629, "format (%.3f)"="%.10f", "1D data"=w624, "append to file? (new file:F)"=TRUE) -> ()  [unwired: 10 in, 2 out]
            n134 = Build Array (concatenate)(w613, w611) -> (w612:dbl[])
          }
          frame #5 {
            n135 = Bundle(w634, w633) -> (→"XY Graph":cluster{dbl[], dbl[]})  [unwired: 1 in]
          }
        }
      }
    }
    frame #4 {
      # "turn off PMT and close"
      n136 = local read "quarter waveplate p1"() -> (w638:dbl)
      n137 = Boolean To (0,1)(Boolean=FALSE) -> (0, 1=w649:i16)
      n138 = To Long Integer(number=w649) -> (32bit integer=w648:i32)
      n139 = call "Set HV.vi"("HV"=w648, "handle"=w644) -> ("handle out"=w646:i32)  [unwired: 8 in, 1 out]
      n140 = invoke class="KCubeDCServo" method="SetMoveAbsolutePosition"(reference=w637, "position"=w638) -> (reference out=w643:refnum<k24>)  [unwired: 2 in, 3 out]
      n141 = call "Read HV.vi"("handle"=w646) -> ("HV out"=w650:i32, "handle out"=w645:i32)  [unwired: 8 in, 1 out]
      n142 = invoke class="KCubeDCServo" method="MoveAbsolute"(reference=w643, "waitTimeout"=0) -> (reference out=w636:refnum<k24>)  [unwired: 2 in, 3 out]
      n143 = invoke class="KCubeDCServo" method="GetPositionCounter"(reference=w636) -> ("GetPositionCounter"=w640:i32)  [unwired: 2 in, 2 out]
      n144 = call "Close.vi"("Handle"=w645) -> ()  [unwired: 9 in, 2 out]
      n145 = local write "PowerD"(w650) -> ()
      n146 = Divide(x=w640, y=1919.6418578623338) -> (x/y=w639:dbl)
      n147 = local write "PC"(w639) -> ()
    }
  }
